vi "Init.vi"(8 "error in (no error)":errorcluster, 11 "appended array":refnum<vi>[][](array[refnum])) -> (0 "error out":errorcluster)   [LabVIEW 2015]
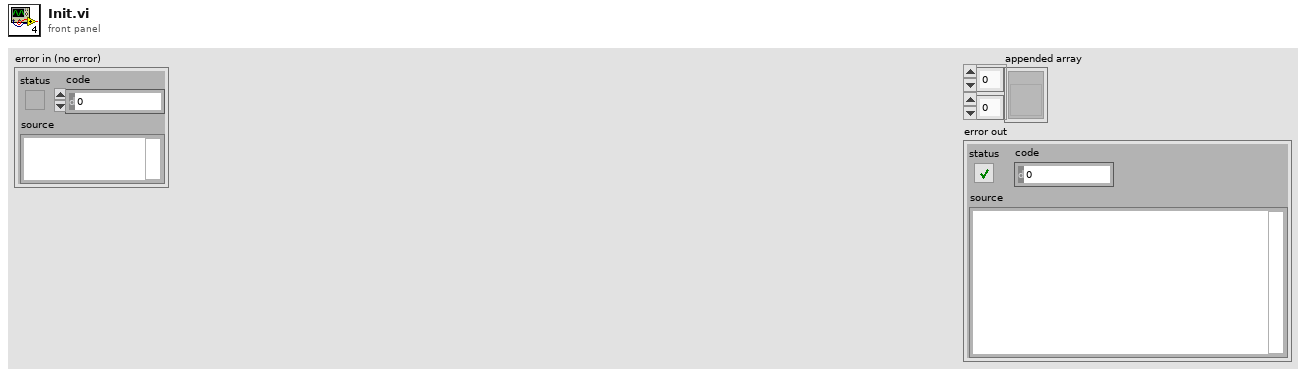
[diagram p1: front panel]
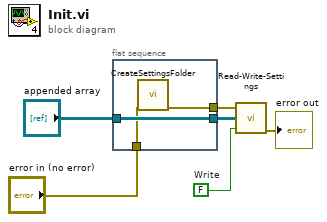
[diagram p0: block diagram]
diagram:
  w5 = FALSE  # Write
  n1 = flat-sequence {
    tunnel: [w9] -> w4
    tunnel: [w8] -> w6
    tunnel: "appended array" -> [w8]
    tunnel: "error in (no error)" -> [w7]
    frame #0 {
      n2 = call "CreateSettingsFolder.vi"("error in (no error)"=w7) -> ("error out"=w9:errorcluster)  [unwired: 10 in]
    }
  }
  n3 = call "Read-Write-Settings.vi"("error in"=w4, "appended array"=w6, "Write"=w5) -> ("error out"=→"error out":errorcluster)  [unwired: 4 in]
